vi "goto.vi"(8 "错误输入（无错误）":errorcluster, 10 "Y(mm)":dbl format="%#_13g", 11 "X(mm)":dbl format="%#_13g") -> (0 "错误输出":errorcluster)   [LabVIEW 2013]
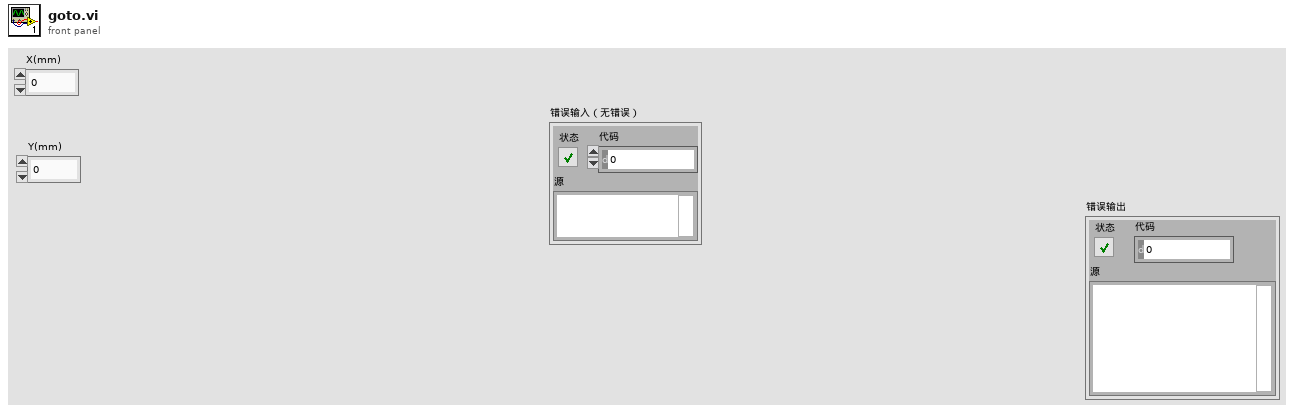
[diagram p1: front panel]
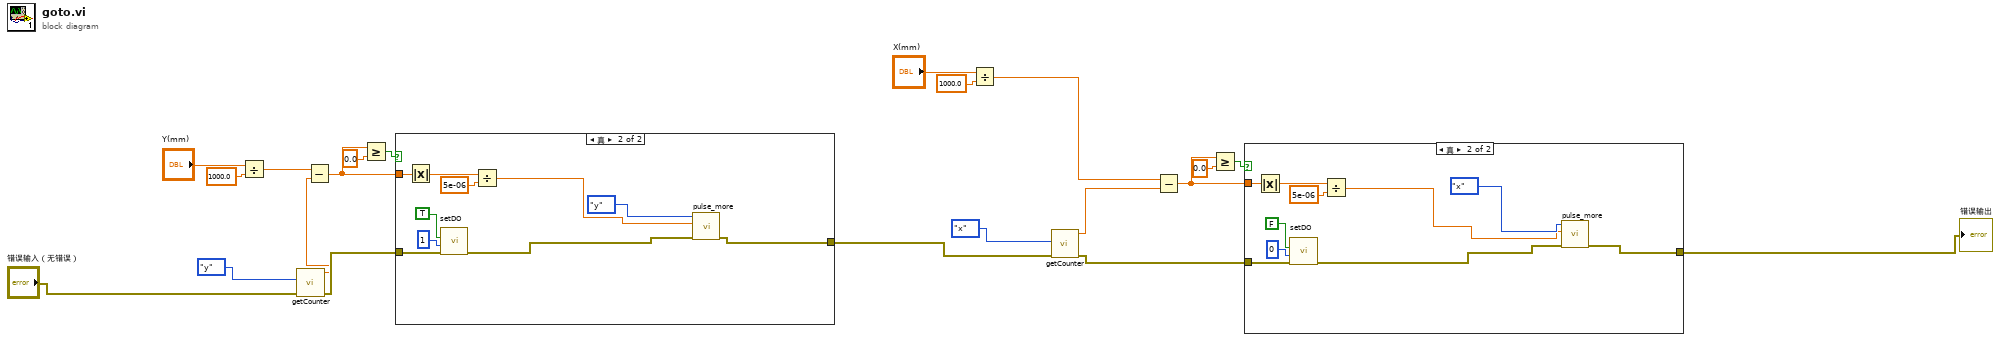
[diagram p0: block diagram]
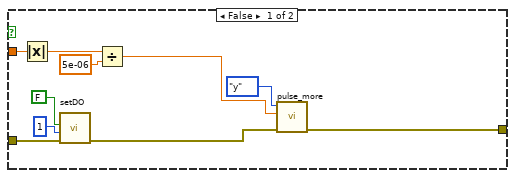
[diagram p2: hidden frame]
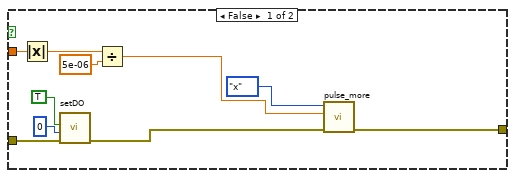
[diagram p3: hidden frame]
diagram:
  n1 = Divide(x="Y(mm)", y=1000.0) -> (x/y=w6:dbl)
  n2 = call "getCounter.vi"("错误输入（无错误）"="错误输入（无错误）", "channel"=enum16{"x", "y"}."y" ("axie")) -> ("错误输出"=w4:errorcluster, "result"=w3:dbl)  [unwired: 8 in]
  n3 = Subtract(x=w6, y=w3) -> (x-y=w9:dbl)
  n4 = Greater Or Equal?(x=w9, y=0.0) -> (x >= y?=w10:bool)
  n5 = case shown="真" w10 {
    tunnel: w9 -> [w25 w35]
    tunnel: w4 -> [w26 w36]
    tunnel: [w23 w33] -> w2
    frame False {
      n6 = Absolute Value(x=w25) -> (abs(x)=w24:dbl)
      n7 = call "setDO.vi"("错误输入（无错误）"=w26, "channel"=1, "on/off"=FALSE) -> ("错误输出"=w22:errorcluster)  [unwired: 8 in]
      n8 = Divide(x=w24, y=5e-06) -> (x/y=w28:dbl)
      n9 = call "pulse_more.vi"("错误输入（无错误）"=w22, "pulse num"=w28, "axie"=enum16{"x", "y"}."y") -> ("错误输出"=w23:errorcluster)  [unwired: 8 in]
    }
    frame True {
      n10 = Absolute Value(x=w35) -> (abs(x)=w34:dbl)
      n11 = call "setDO.vi"("错误输入（无错误）"=w36, "channel"=1, "on/off"=TRUE) -> ("错误输出"=w32:errorcluster)  [unwired: 8 in]
      n12 = Divide(x=w34, y=5e-06) -> (x/y=w38:dbl)
      n13 = call "pulse_more.vi"("错误输入（无错误）"=w32, "pulse num"=w38, "axie"=enum16{"x", "y"}."y") -> ("错误输出"=w33:errorcluster)  [unwired: 8 in]
    }
  }
  n14 = Divide(x="X(mm)", y=1000.0) -> (x/y=w16:dbl)
  n15 = call "getCounter.vi"("错误输入（无错误）"=w2, "channel"=enum16{"x", "y"}."x" ("axie")) -> ("错误输出"=w15:errorcluster, "result"=w13:dbl)  [unwired: 8 in]
  n16 = Subtract(x=w16, y=w13) -> (x-y=w19:dbl)
  n17 = Greater Or Equal?(x=w19, y=0.0) -> (x >= y?=w20:bool)
  n18 = case shown="真" w20 {
    tunnel: w19 -> [w45 w57]
    tunnel: w15 -> [w46 w58]
    tunnel: [w43 w55] -> w12
    frame False {
      n19 = Absolute Value(x=w45) -> (abs(x)=w44:dbl)
      n20 = call "setDO.vi"("错误输入（无错误）"=w46, "channel"=0, "on/off"=TRUE) -> ("错误输出"=w42:errorcluster)  [unwired: 8 in]
      n21 = Divide(x=w44, y=5e-06) -> (x/y=w48:dbl)
      n22 = call "pulse_more.vi"("错误输入（无错误）"=w42, "pulse num"=w48, "axie"=enum16{"x", "y"}."x") -> ("错误输出"=w43:errorcluster)  [unwired: 8 in]
    }
    frame True {
      n23 = Absolute Value(x=w57) -> (abs(x)=w56:dbl)
      n24 = call "setDO.vi"("错误输入（无错误）"=w58, "channel"=0, "on/off"=FALSE) -> ("错误输出"=w52:errorcluster)  [unwired: 8 in]
      n25 = Divide(x=w56, y=5e-06) -> (x/y=w53:dbl)
      n26 = call "pulse_more.vi"("错误输入（无错误）"=w52, "pulse num"=w53, "axie"=enum16{"x", "y"}."x") -> ("错误输出"=w55:errorcluster)  [unwired: 8 in]
    }
  }
  "错误输出" <- w12
